vi "项操作.vi"(8 "error in (no error)":errorcluster caption="错误输入（无错误）", 9 "Cell Position":T1, 10 "MCListbox引用句柄":refnum<vi>, 11 "LNK 输入":refnum<class "Down.lvclass">) -> (0 "error out":errorcluster caption="错误输出", 3 "LNK 输出":refnum<class "Down.lvclass">)   [LabVIEW 2016, in "Down.lvclass"]
uses:
  Down.lvclass
  <vilib>/Utility/miscctls.llb/LVRowAndColumnTypeDef.ctl
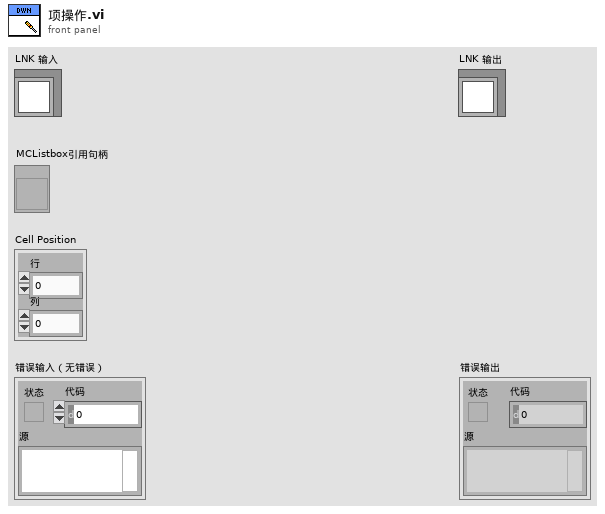
[diagram p1: front panel]
types:
  T1 = typedef "LVRowAndColumnTypeDef.ctl" = cluster{"Row":i32, "Column":i32}
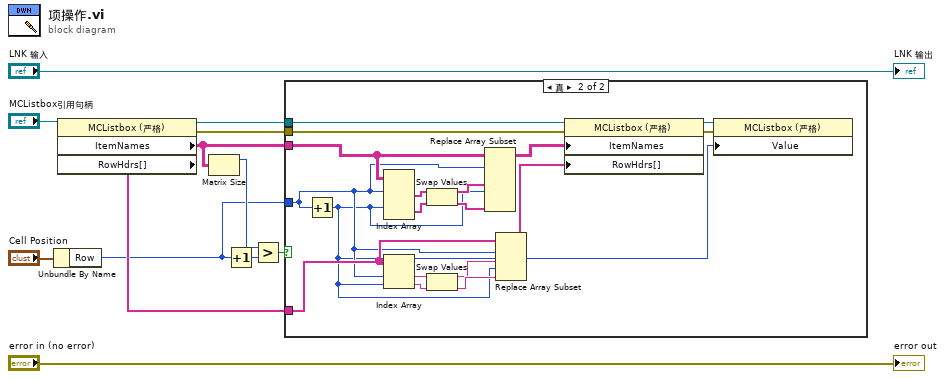
[diagram p0: block diagram]
diagram:
  n1 = Unbundle By Name("Cell Position") -> ("Row"=w1:i32)
  n2 = property class="MCListbox (严格)"(reference="MCListbox引用句柄") -> (reference out=w9:refnum<vi>, error out=w10:errorcluster, "ItemNames"=w7:string[][], "RowHdrs[]"=w3:string[])  [unwired: 1 in]
  n3 = Matrix Size(0:w7) -> (1:w6:i32)  [unwired: 1 out]
  n4 = Increment(x=w1) -> (x+1=w4:i32)
  n5 = Greater?(x=w6, y=w4) -> (0:w5:bool)
  n6 = case shown="真" w5 {
    tunnel: w9 -> [_ w30]
    tunnel: w10 -> [_ w29]
    tunnel: w7 -> [_ w28]
    tunnel: w1 -> [_ w14]
    tunnel: w3 -> [_ w15]
    frame False {
    }
    frame True {
      n7 = Increment(x=w14) -> (x+1=w13:i32)
      n8 = Index Array(array=w28, index (row) #1=w14, index (row) #2=w13) -> (element #1=w24:string[], element #2=w22:string[])  [unwired: 2 in]
      n9 = Index Array(array=w15, index #1=w14, index #2=w13) -> (element #1=w17:string, element #2=w19:string)
      n10 = Swap Values(12:w24, 14:w22) -> (1:w23:string[], 3:w21:string[])  [unwired: 1 in]
      n11 = Swap Values(12:w17, 14:w19) -> (1:w18:string, 3:w20:string)  [unwired: 1 in]
      n12 = Replace Array Subset(array=w28, new element #1=w23, index (row) #1=w14, new element #2=w21, index (row) #2=w13) -> (w27:string[][])  [unwired: 2 in]
      n13 = Replace Array Subset(array=w15, new element #1=w18, index #1=w14, new element #2=w20, index #2=w13) -> (w16:string[])
      n14 = property class="MCListbox (严格)"(reference=w30, error in=w29, "ItemNames"=w27, "RowHdrs[]"=w16) -> (reference out=w26:refnum<vi>, error out=w25:errorcluster)
      n15 = property class="MCListbox (严格)"(reference=w26, error in=w25, "Value"=w13) -> ()  [unwired: 2 out]
    }
  }
  "error out" <- "error in (no error)"
  "LNK 输出" <- "LNK 输入"
